vi "APP_FileWriter.vi"(0 "path (use dialog)":path, 1 "input byte stream":u8[](array[numeric])) -> (7 "path":path)   [LabVIEW 2014]
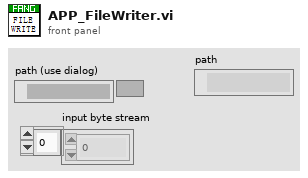
[diagram p1: front panel]
types:
  T1 = enum16{"open", "replace", "create", "open or create", "replace or create", "replace or create with confirmation"}
  T2 = enum16{"big-endian, network order", "native, host order", "little-endian"}
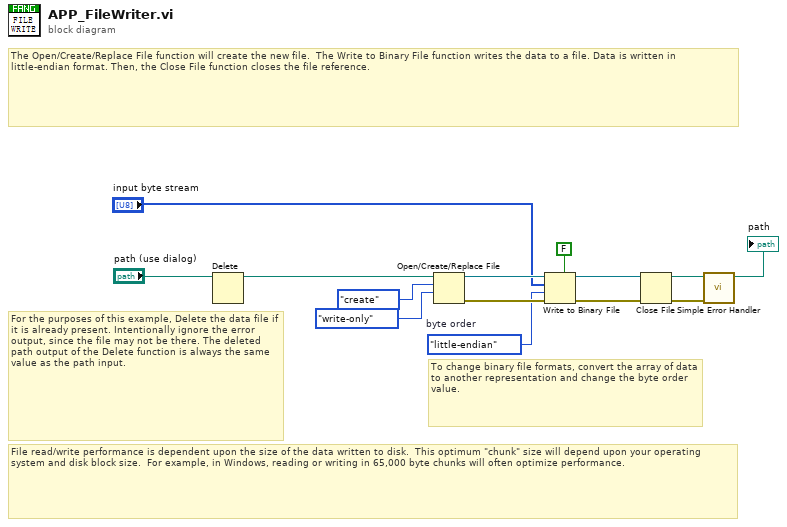
[diagram p0: block diagram]
diagram:
  w6 = T2."little-endian"  # byte order
  # "File read/write performance is dependent upon the size of the data written to disk.  This optimum \"chunk\" size will depend upon your operating system and disk block size.  For example, in Windows, reading or writing in 65,000 byte chunks will often optimize performance."
  # "To change binary file formats, convert the array of data to another representation and change the byte order value."
  # "For the purposes of this example, Delete the data file if it is already present. Intentionally ignore the error output, since the file may not be there. The deleted path output of the Delete function is always the same value as the path input."
  # "The Open/Create/Replace File function will create the new file.  The Write to Binary File function writes the data to a file. Data is written in little-endian format. Then, the Close File function closes the file reference."
  n1 = Delete(path (use dialog)="path (use dialog)") -> (deleted path=w4:path)  [unwired: 4 in, 2 out]
  n2 = Open/Create/Replace File(file path (use dialog)=w4, operation (0:open)=T1."create", access (0:read/write)=enum16{"read/write", "read-only", "write-only"}."write-only") -> (refnum out=w9:refnum<file>, error out=w10:errorcluster)  [unwired: 3 in, 1 out]
  n3 = Write to Binary File(file (use dialog)=w9, data="input byte stream", error in=w10, 5:FALSE ("prepend array or string size? (T)"), 9:w6) -> (refnum out=w13:refnum<file>, error out=w12:errorcluster)  [unwired: 1 in, 1 out]
  n4 = Close File(refnum=w13, error in=w12) -> (path=→"path":path, error out=w11:errorcluster)
  n5 = call <vilib>:"Simple Error Handler.vi"("error in (no error)"=w11) -> ()  [unwired: 4 in, 5 out]
